vi "compute_statistics_data_starter.vi"() -> ()   [LabVIEW 2018]
uses:
  Controls/StatisticsData.ctl
  Classes/Phase/Phase.lvclass
  Classes/HasoSlopes/HasoSlopes.lvclass
  Controls/WavefrontReconstructionMode.ctl
  Classes/Pupil/Pupil.lvclass
panel:
  out "Wavefront":sgl[][](graph)
  in  "Haso slopes file name":string="Data\\data_phase_computation.has"
  out "error out":errorcluster
  out "Statistics":T1
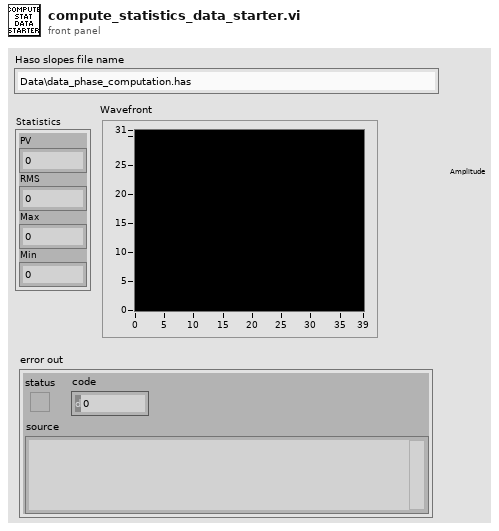
[diagram p1: front panel]
types:
  T1 = typedef "StatisticsData.ctl" = cluster{"PV":sgl, "RMS":dbl, "Max":sgl, "Min":sgl}
  T2 = typedef "WavefrontReconstructionMode.ctl" = enum16{"None", "Modal_Legendre", "Modal_Zernike", "Zonal", "Modal_Zonal_Zernike", "Modal_Zonal_Legendre"}
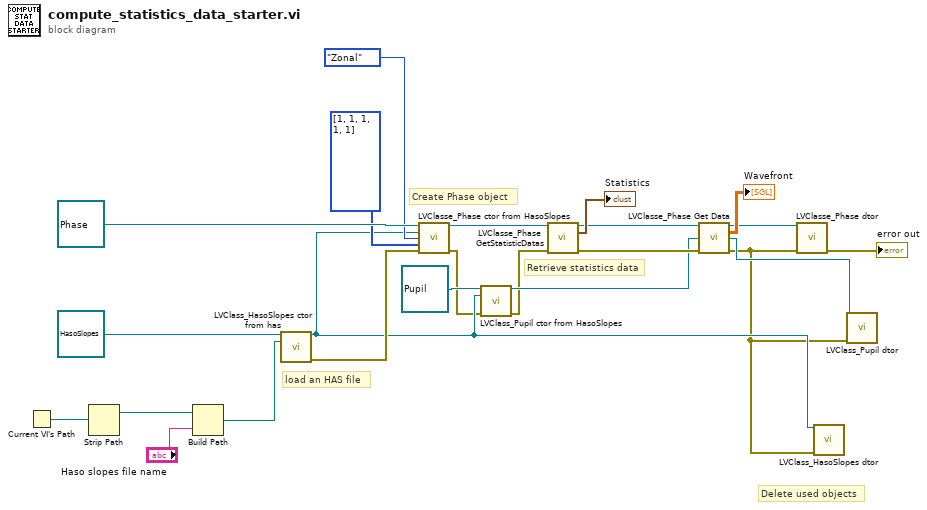
[diagram p0: block diagram]
diagram:
  # "Retrieve statistics data"
  # "Create Phase object"
  # "load an HAS file"
  # "Delete used objects"
  n1 = Current VI's Path() -> (path=w22:path)
  n2 = Strip Path(path=w22) -> (stripped path=w20:path)  [unwired: 1 out]
  n3 = Build Path(base path=w20, name or relative path="Haso slopes file name") -> (appended path=w12:path)
  n4 = call "LVClass_HasoSlopes ctor from has.vi"("HasoSlopes (const)"=refnum<class "HasoSlopes.lvclass"> refnum ("HasoSlopes in"), ".has path"=w12) -> ("HasoSlopes (new)"=w6:refnum<class "HasoSlopes.lvclass">, "error out"=w16:errorcluster)  [unwired: 12 in]
  n5 = call "LVClasse_Phase ctor from HasoSlopes.vi"("Phase (const)"=refnum<class "Phase.lvclass"> refnum ("Phase in"), "HasoSlopes"=w6, "TypePhase"=WavefrontReconstructionMode."Zonal", "Filter"=u8[] [1, 1, 1, 1, 1], "error in (no error)"=w16) -> ("Phase (new)"=w13:refnum<class "Phase.lvclass">, "error out"=w2:errorcluster)  [unwired: 8 in, 1 out]
  n6 = call "LVClass_Pupil ctor from HasoSlopes.vi"("Pupil (const)"=refnum<class "Pupil.lvclass"> refnum ("Pupil in"), "HasoSlopes"=w6, "error in (no error)"=w2) -> ("Pupil (new)"=w5:refnum<class "Pupil.lvclass">, "error out"=w1:errorcluster)  [unwired: 10 in, 1 out]
  n7 = call "LVClasse_Phase GetStatisticDatas.vi"("Phase in"=w13, "error in (no error)"=w1) -> ("Phase out"=w10:refnum<class "Phase.lvclass">, "StatisticsData"=→"Statistics":T1, "error out"=w9:errorcluster)  [unwired: 11 in]
  n8 = call "LVClasse_Phase Get Data.vi"("Phase in"=w10, "Pupil"=w5, "error in (no error)"=w9) -> ("Phase out"=w8:refnum<class "Phase.lvclass">, "data"=→"Wavefront":sgl[][], "Pupil (dup)"=w4:refnum<class "Pupil.lvclass">, "error out"=w3:errorcluster)  [unwired: 9 in]
  n9 = call "LVClasse_Phase dtor.vi"("Phase in"=w8, "error in (no error)"=w3) -> ("error out"=→"error out":errorcluster)  [unwired: 12 in, 1 out]
  n10 = call "LVClass_HasoSlopes dtor.vi"("HasoSlopes in"=w6, "error in (no error)"=w3) -> ()  [unwired: 12 in, 2 out]
  n11 = call "LVClass_Pupil dtor.vi"("Pupil in"=w4, "error in (no error)"=w3) -> ()  [unwired: 12 in, 2 out]
